vi "Kommando unique.vi"(9 "remove":bool, 10 "Kommando in (Eingang)":T1, 11 "Array (Eingang)":T1[](array[typedef])) -> (1 "found":bool, 2 "Kommando out":T1, 3 "Array (Ausgang)":T1[](array[typedef]))   [LabVIEW 2020, in "Linearisierung v2.lvlib" / "Gasteiler.lvlib" / "HovaCAL_Interface.lvlib" / "Kommunikation.lvlib"]
uses:
  Kommunikation.lvlib
  Aktion_FGV_HovaCAL_Interface_Kommunikation.ctl
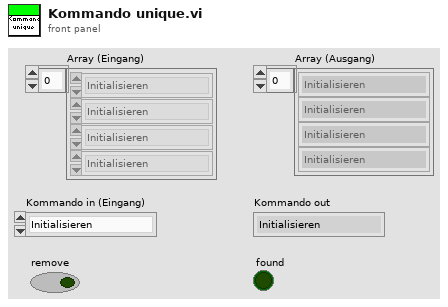
[diagram p1: front panel]
types:
  T1 = typedef "Linearisierung v2.lvlib/Gasteiler.lvlib/HovaCAL_Interface.lvlib/Kommunikation.lvlib/Aktion_FGV_HovaCAL_Interface_Kommunikation.ctl" = enum16{"Initialisieren", "Set Konzentrationen", "Set Gase", "Set Limits", "Get Dynamische Werte", "Beenden", "Com ändern", "Get Gase init", "Pause", "Get Gasteiler Infos", "Get MFC Infos", "Set Pumpen Parameter", "Set Pumpe Konzenration", "Set Pumpe run", "Set Temperaturen", "Set Fluss", "Get Gase", "Get Limits", "Get Dynamische Werte 1", "Get Dynamische Werte 2"}
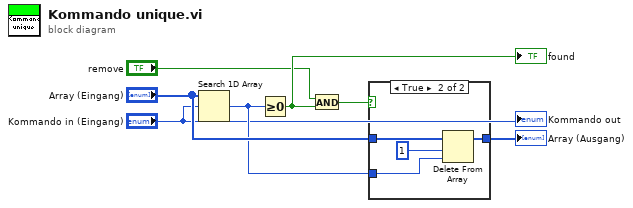
[diagram p0: block diagram]
diagram:
  n1 = Search 1D Array(1D array="Array (Eingang)", element="Kommando in (Eingang)") -> (index of element=w5:i32)  [unwired: 1 in]
  n2 = Greater Or Equal To 0?(x=w5) -> (x >= 0?=w3:bool)
  "found" <- w3
  n3 = And(x="remove", y=w3) -> (x .and. y?=w2:bool)
  n4 = case shown="True" w2 {
    tunnel: [w8 w12] -> w7
    tunnel: "Array (Eingang)" -> [w8 w11]
    tunnel: w5 -> [_ w10]
    frame False {
    }
    frame True {
      n5 = Delete From Array(array=w11, length=1 ("Länge"), index=w10) -> (array with subset deleted=w12:T1[])  [unwired: 1 out]
    }
  }
  "Array (Ausgang)" <- w7
  "Kommando out" <- "Kommando in (Eingang)"
